vi "Request Image.vi"(8 "error in (no error)":errorcluster, 9 "Enqueuer":refnum<class "Message Enqueuer.lvclass">, 10 "Image Acquisition.lvlib:Image Msg.lvclass":refnum<class "Image Msg.lvclass">, 11 "Controller in":refnum<class "Controller.lvclass">) -> (0 "error out":errorcluster, 3 "Controller out":refnum<class "Controller.lvclass">)   [LabVIEW 2016, in "Controller.lvlib" / "Controller.lvclass"]
uses:
  Controller.lvclass
  Image Acquisition/Image Acquisition Messages/Image Msg/Image Msg.lvclass
  <vilib>/ActorFramework/Message Enqueuer/Message Enqueuer.lvclass
  Controller.lvclass/Controller.ctl
  Image Acquisition/Image Acquisition Messages/Request For Image Msg/Request For Image Msg.lvclass/Request For Image Msg.ctl
  <vilib>/ActorFramework/Message Enqueuer/Message Enqueuer.lvclass/Message Enqueuer.ctl
  <vilib>/ActorFramework/Message Enqueuer/Enqueue.vi
  Image Acquisition/Image Acquisition Messages/Request For Image Msg/Request For Image Msg.lvclass
  C:/Program Files (x86)/National Instruments/LabVIEW 2016/vi.lib/ActorFramework/Message/Message.lvclass
  <vilib>/ActorFramework/Message Priority Queue/Priority Enqueue.vi
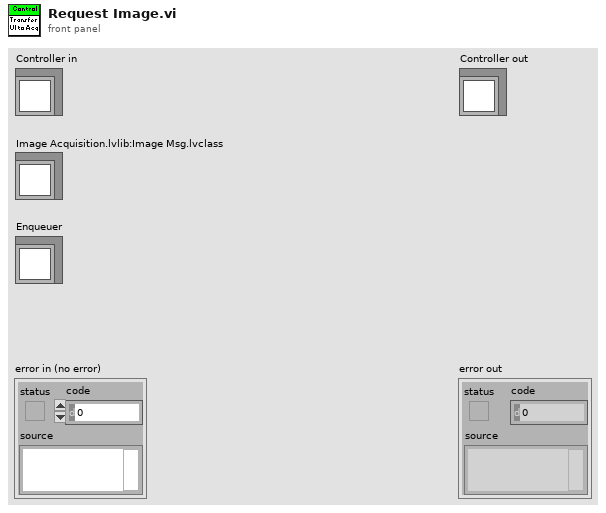
[diagram p1: front panel]
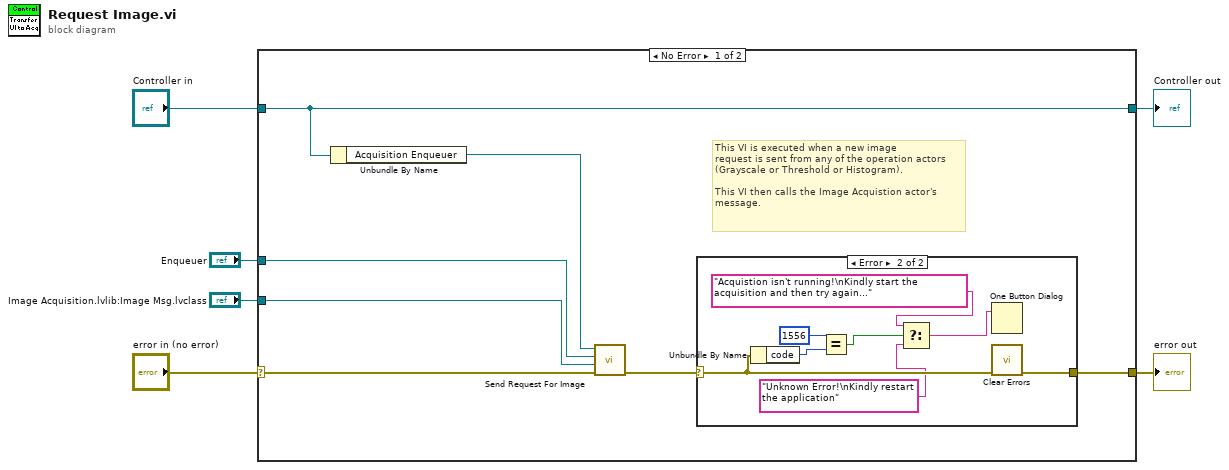
[diagram p0: block diagram]
diagram:
  n1 = case shown="No Error" "error in (no error)" {
    selector: "error in (no error)" -> [w12 w24]
    tunnel: [w7 w24] -> w5
    tunnel: [w13 w23] -> w3
    tunnel: "Controller in" -> [w13 w23]
    tunnel: "Image Acquisition.lvlib:Image Msg.lvclass" -> [w9 _]
    tunnel: "Enqueuer" -> [w10 _]
    frame No Error {
      # "This VI is executed when a new image\nrequest is sent from any of the operation actors\n(Grayscale or Threshold or Histogram).\n\nThis VI then calls the Image Acquistion actor's\nmessage."
      n2 = Unbundle By Name(w13) -> ("Acquisition Enqueuer"=w11:refnum<class "Message Enqueuer.lvclass">)
      n3 = call "Send Request For Image.vi"("error in (no error)"=w12, "Caller Messge"=w9, "Caller Enqueuer"=w10, "Message Enqueuer"=w11) -> ("error out"=w8:errorcluster)  [unwired: 6 in, 1 out]
      n4 = case shown="Error" w8 {
        selector: w8 -> [w14 w21]
        tunnel: [w14 w22] -> w7
        frame No Error {
        }
        frame Error {
          n5 = Unbundle By Name(w21) -> ("code"=w20:i32)
          n6 = Equal?(x=1556, y=w20) -> (x = y?=w18:bool)
          n7 = Select(t="Acquistion isn't running!\nKindly start the acquisition and then try again..." ("message"), s=w18, f="Unknown Error!\nKindly restart the application" ("message")) -> (s? t:f=w15:string)
          n8 = One Button Dialog(message=w15) -> ()  [unwired: 1 in, 1 out]
          n9 = call <vilib>:"Clear Errors.vi"("error in (no error)"=w21) -> ("error out"=w22:errorcluster)  [unwired: 5 in, 1 out]
        }
      }
    }
    frame Error {
    }
  }
  "error out" <- w5
  "Controller out" <- w3
